vi "Field Draw Future Robots.vi"(4 "Lado":enum16{"Esquerdo", "Direito"}(ring) caption="Enum", 6 "Draw Targets?":T1, 7 "RobotRef":refnum<class "Robot.lvclass">[](array[class]), 8 "Offset":cluster{"Width":dbl, "Height":dbl}, 9 "Picture In":picture, 10 "Scale":dbl) -> (0 "Picture Out":picture, 1 "Offset Out":cluster{"Width":dbl, "Height":dbl}, 2 "Scale Out":dbl)   [LabVIEW 2023]
uses:
  DrawTargets.ctl
  Robot_class/Robot.lvclass
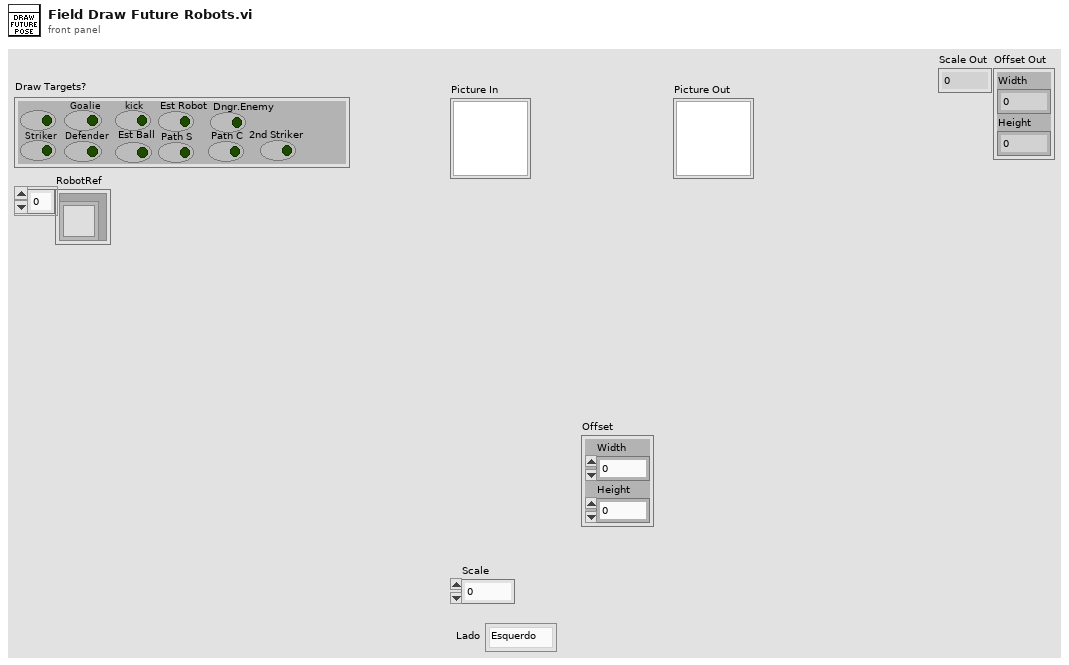
[diagram p1: front panel]
types:
  T1 = typedef "DrawTargets.ctl" = cluster{"Attacker":bool, "Striker":bool, "Goalie":bool, "Defender":bool, "kick":bool, "Est Ball":bool, "Est Robot":bool, "Path S":bool, "Path C":bool, "Dngr.Enemy":bool, "2nd Striker":bool}
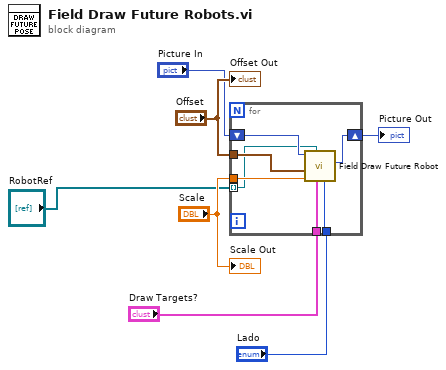
[diagram p0: block diagram]
diagram:
  n1 = for {
    tunnel: "Scale" -> [w11]
    tunnel: "Offset" -> [w14]
    shift-right: [w13] -> w4
    shift-left: "Picture In" -> [w12]
    tunnel: "Draw Targets?" -> [w10]
    tunnel: "Lado" -> [w9]
    tunnel: "RobotRef" -> [w8] mode=indexing
    n2 = call "Field Draw Future Robot.vi"("Lado"=w9, "Draw Targets?"=w10, "Robot 2"=w8, "Scale mm/pixel"=w11, "Offset"=w14, "picture in"=w12) -> ("picture out"=w13:picture)  [unwired: 5 in]
  }
  "Picture Out" <- w4
  "Scale Out" <- "Scale"
  "Offset Out" <- "Offset"
